vi "Stop.vi"(6 "Teller":T1 {"AbsoluteTime" format="%<%x %.3X>T"}, 8 "Error in":errorcluster, 11 "Base Actor in":refnum<class "Base Actor.lvclass">) -> (0 "Error out":errorcluster, 3 "Base Actor out":refnum<class "Base Actor.lvclass">)   [LabVIEW 2020, in "jettl.lvlib" / "BaseActor.lvlib" / "Base Actor.lvclass"]
uses:
  Base Actor.lvclass
  Base Actor.lvclass/Base Actor.ctl
  jettl.lvlib
  ActorLifetime.ctl
  ActorRelation.ctl
  MessageMetadata.ctl
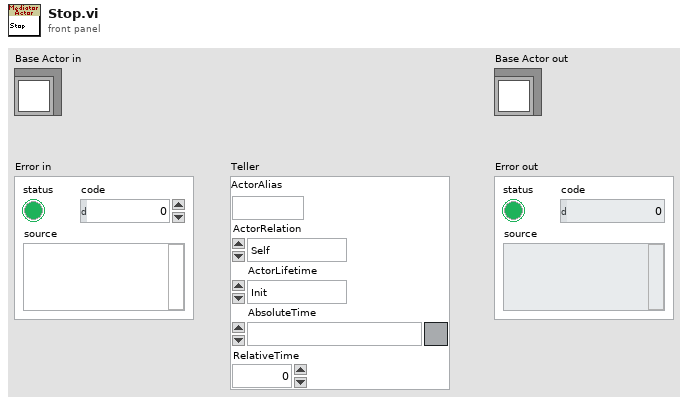
[diagram p1: front panel]
types:
  T1 = typedef "jettl.lvlib/MessageMetadata.ctl" = cluster{"ActorAlias":string, "ActorRelation":T2, "ActorLifetime":T3, "AbsoluteTime":timestamp, "RelativeTime":dbl}
  T2 = typedef "jettl.lvlib/ActorRelation.ctl" = enum16{"Self", "Mediator", "Component"}
  T3 = typedef "jettl.lvlib/ActorLifetime.ctl" = enum16{"Init", "Spawn", "Setup", "Teardown Before Running", "Running", "Stop Called", "Stopping With Children", "Stopping Without Children", "Teardown After Running", "Stopped"}
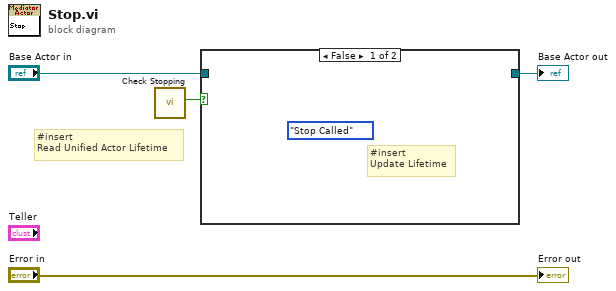
[diagram p0: block diagram]
diagram:
  # "#insert\nRead Unified Actor Lifetime"
  n1 = call "Check Stopping.vi"() -> ("Stopping"=w3:bool, "Unified Actor Lifetime"=w1:T3)  [unwired: 10 in]
  n2 = case shown="False" w3 {
    tunnel: "Base Actor in" -> [w7 w9]
    tunnel: [w6 w9] -> w4
    frame False {
      w8 = ActorLifetime."Stop Called" ("Lifetime")
      # "#insert\nUpdate Lifetime"
    }
    frame True {
    }
  }
  "Base Actor out" <- w4
  "Error out" <- "Error in"
